vi "ControlDtcSetting.vi"(5 "LogSuspend":bool, 8 "error in":errorcluster, 10 "Subfunction":enum8{"ON", "OFF"}(ring), 11 "UdsHandleIn":T1={"LogPath"=path "", "LogEnabled"=FALSE, "isOpen"=FALSE, "LogContent"="", "Adapter"="CAN0", "MCanHandle"={"MCanAdapter"=refnum}, "TransmittId"=0, "ReceiveId"=0}) -> (0 "error out":errorcluster, 3 "UdsHandleOut":T1={"LogPath"=path "", "LogEnabled"=FALSE, "isOpen"=FALSE, "LogContent"="", "Adapter"="CAN0", "MCanHandle"={"MCanAdapter"=refnum}, "TransmittId"=0, "ReceiveId"=0})   [LabVIEW 2011, in "Konvolucio MUDS150628.lvlib"]
uses:
  <instrlib>/Konvolucio MUDS150628/Konvolucio MUDS150628.lvlib
  <instrlib>/Konvolucio MUDS150628/Types/UdsHandleType.ctl
  <instrlib>/Konvolucio MCAN120803/Types/MCanHandleType.ctl
  C:/Program Files/National Instruments/LabVIEW 2011/instr.lib/Konvolucio MCAN120803/Private/Konvolucio.MCAN120803.dll
  Konvolucio MCAN120803/Private/Konvolucio.MCAN120803.dll
  <instrlib>/Konvolucio MCAN120803/Konvolucio MCAN120803.lvlib
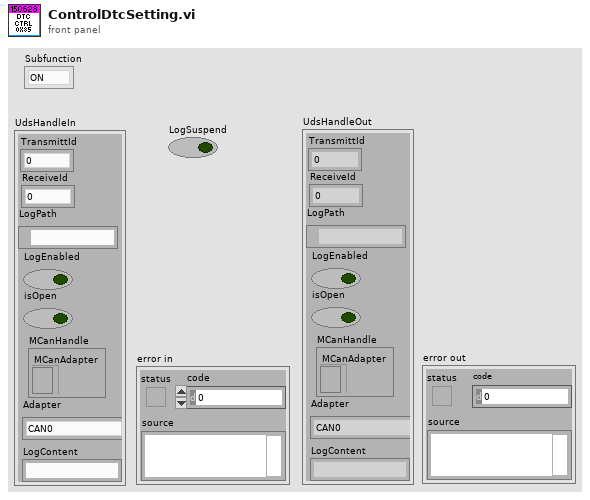
[diagram p1: front panel]
types:
  T1 = typedef "Konvolucio MUDS150628.lvlib/UdsHandleType.ctl" = cluster{"LogPath":path, "LogEnabled":bool, "isOpen":bool, "LogContent":string, "Adapter":string, "MCanHandle":T2, "TransmittId":u32, "ReceiveId":u32}
  T2 = typedef "Konvolucio MCAN120803.lvlib/MCanHandleType.ctl" = cluster{"MCanAdapter":refnum<k24>}
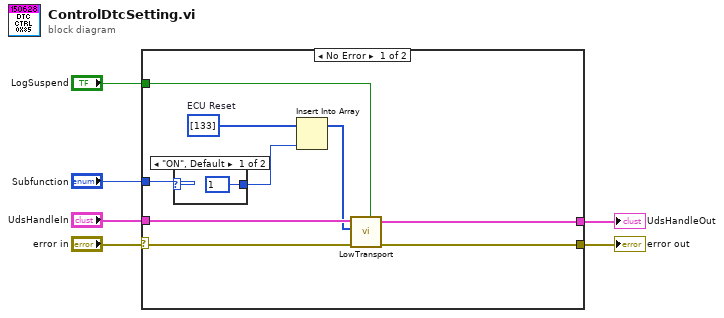
[diagram p0: block diagram]
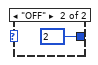
[diagram p2: hidden frame]
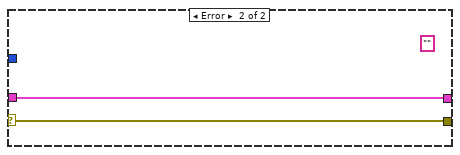
[diagram p3: hidden frame]
diagram:
  n1 = case shown="No Error" "error in" {
    selector: "error in" -> [w14 w19]
    tunnel: "UdsHandleIn" -> [w15 w18]
    tunnel: [w13 w19] -> w4
    tunnel: [w12 w18] -> w3
    tunnel: "LogSuspend" -> [w11 _]
    tunnel: "Subfunction" -> [w8 _]
    frame No Error {
      w10 = u8[] [133]  # ECU Reset
      n2 = case shown="\"ON\", Default" w8 {
        tunnel: [1 2] -> w7
        frame "ON", Default {
        }
        frame "OFF" {
        }
      }
      n3 = Insert Into Array(array=w10, new element=w7) -> (w9:u8[])  [unwired: 1 in]
      n4 = call <instrlib>:"LowTransport.vi"("LogSuspend"=w11, "error in"=w14, "Request"=w9, "HandleIn"=w15) -> ("error out"=w13:errorcluster, "HandleOut"=w12:T1)  [unwired: 5 in, 1 out]
    }
    frame Error {
      (unwired) "" ("HexStringArrayOut")
    }
  }
  "error out" <- w4
  "UdsHandleOut" <- w3
